vi "Write INI Cluster__ogtk.vi"(5 "float number format (optional)":string, 8 "error in (no error)":errorcluster, 10 "INI Fomatted Cluster":variant, 11 "refnum":T1) -> (0 "error out":errorcluster, 3 "dup refnum":T1)   [LabVIEW 2017]
doc: "Writes a cluster of section formatted clusters to configuration data identified by refnum. Section cluster names are used as section names and key-value pairs correspond to the named cluster elements and thier values within the section formatted clusters. Only the items within the \"INI Formatted Cluster\" input cluster are written to the configuration data.\n\nFor example an Cluster containins subClusters MyCluster1 and MyCluster2, where MyCluster1 contains two elements MyNumeric and MyBoolean, and MyCluster2 contains two elements MyEnum and MyString. This would correspond to an INI write of the following data:\n\n[MyCluster1]\nMyNumeric=1.024\nMyBoolean=TRUE\n[MyCluster2]\nMyEnum=init\nMyString=\"Hello World\"\n\nNote: Special characters in section and key names will be escape-coded. These include the following: \\00-\\1F (non-printable chars); \"[\", \"]\", and \"=\" (INI syntax elements); \\FE (\"þ\") and \\FF (\"ÿ\") (legacy bracket encoding); Additionally, the escape character, \"\\\", will be escaped as \"\\\\\".\n\nNote: This VI checks whether every element of the cluster has a name so it can be identified."
uses:
  <vilib>/Utility/config.llb/Config Data RefNum.ctl
  <vilib>/Utility/config.llb/NI_LVConfig.lvlib
panel:
  # "Write INI Cluster.vi\n\nWrites a cluster (variant) of INI section clusters to INI file.\n\nPlease visit http://www.OpenG.org to learn about the\nOpen Source LabVIEW software movement.\n\nNOTICE -- YOU MUST LEAVE THIS NOTICE IN PLACE.  PER THE TERMS OF THE LICENSE BELOW, YOU MAY SUBLICENSE THIS SOFTWARE \nIN ANY WAY THAT DOES NOT CONFLICT WITH THIS LICENSE.\n\n### BSD License (http://www.opensource.org/licenses/bsd-license.php) Begin ###\n \nCopyright (c) 2002-2006, Jim Kring <jim@jimkring.com>\n\nAll rights reserved.\n\nRedistribution and use in source and binary forms, with or without modification, are permitted provided that the following conditions are met:\n\n    * Redistributions of source code must retain the above copyright notice, this list of conditions and the following disclaimer.\n    * Redistributions in binary form must reproduce the above copyright notice, this list of conditions and the following disclaimer in the \n       documentation and/or other materials provided with the distribution.\n    * Neither the name of SciWare, James Kring, Inc., nor the names of its contributors may be used to endorse or promote products derived \n       from this software without specific prior written permission.\n\nTHIS SOFTWARE IS PROVIDED BY THE COPYRIGHT HOLDERS AND CONTRIBUTORS \"AS IS\" AND ANY EXPRESS OR IMPLIED WARRANTIES, \nINCLUDING, BUT NOT LIMITED TO, THE IMPLIED WARRANTIES OF MERCHANTABILITY AND FITNESS FOR A PARTICULAR PURPOSE ARE \nDISCLAIMED. IN NO EVENT SHALL THE COPYRIGHT OWNER OR CONTRIBUTORS BE LIABLE FOR ANY DIRECT, INDIRECT, INCIDENTAL,\n SPECIAL, EXEMPLARY, OR CONSEQUENTIAL DAMAGES (INCLUDING, BUT NOT LIMITED TO, PROCUREMENT OF SUBSTITUTE GOODS OR \nSERVICES; LOSS OF USE, DATA, OR PROFITS; OR BUSINESS INTERRUPTION) HOWEVER CAUSED AND ON ANY THEORY OF LIABILITY, \nWHETHER IN CONTRACT, STRICT LIABILITY, OR TORT (INCLUDING NEGLIGENCE OR OTHERWISE) ARISING IN ANY WAY OUT OF THE USE \nOF THIS SOFTWARE, EVEN IF ADVISED OF THE POSSIBILITY OF SUCH DAMAGE.\n\n### BSD License End ###"
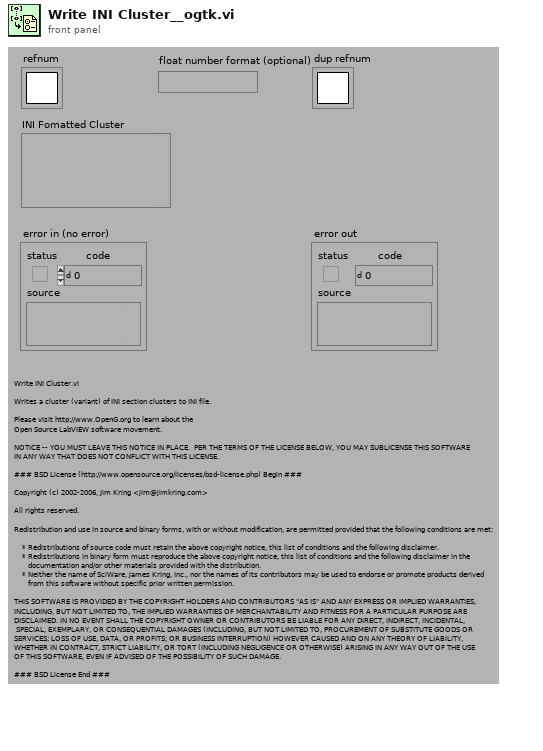
[diagram p1: front panel]
types:
  T1 = typedef "NI_LVConfig.lvlib/Config Data RefNum.ctl" = refnum<k1>
  T2 = typedef "Type Descriptor Enumeration__ogtk.ctl" = enum8{"<Null>", "I8", "I16", "I32", "I64", "U8", "U16", "U32", "U64", "SGL", "DBL", "EXT", "CSG", "CDB", "CXT", "0x0F", "0x10", "0x11", "0x12", "0x13", "0x14", "Enum U8", "Enum U16", "Enum U32", "Enum U64", "SGL PQ", "DBL PQ", "EXT PQ", "CSG PQ", "CDB PQ", "CXT PQ", "0x1F", "0x20", "Boolean", "0x22", "0x23", "0x24", "0x25", "0x26", "0x27", "0x28", "0x29", "0x2A", "0x2B", "0x2C", "0x2D", "0x2E", "0x2F", "String", "0x31", "Path", "Pict", "0x34", "0x35", "0x36", "DAQ", "0x38", "0x39", "0x3A", "0x3B", "0x3C", "0x3D", "0x3E", "0x3F", "Array", "0x41", "0x42", "0x43", "0x44", "0x45", "0x46", "0x47", "0x48", "0x49", "0x4A", "0x4B", "0x4C", "0x4D", "0x4E", "0x4F", "Cluster", "0x51", "0x52", "Variant", "Waveform", "0x55", "0x56", "0x57", "0x58", "0x59", "0x5A", "0x5B", "0x5C", "0x5D", "0x5E", "0x5F", "0x60", "0x61", "0x62", "0x63", "0x64", "0x65", "0x66", "0x67", "0x68", "0x69", "0x6A", "0x6B", "0x6C", "0x6D", "0x6E", "0x6F", "Refnum"}
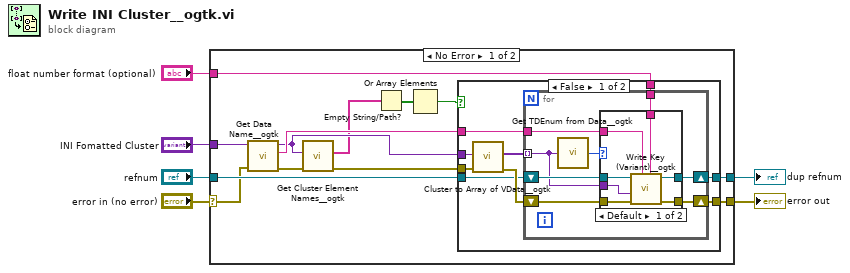
[diagram p0: block diagram]
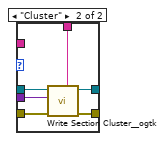
[diagram p2: hidden frame]
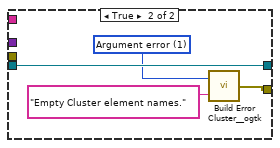
[diagram p3: hidden frame]
diagram:
  n1 = case shown="No Error" "error in (no error)" {
    selector: "error in (no error)" -> [w14 w55]
    tunnel: [w19 w55] -> w6
    tunnel: [w18 w54] -> w5
    tunnel: "refnum" -> [w17 w54]
    tunnel: "INI Fomatted Cluster" -> [w16 _]
    tunnel: "float number format (optional)" -> [w15 _]
    frame No Error {
      n2 = call <userlib>:"Get Data Name__ogtk.vi"("error in (no error)"=w14, "Data"=w16) -> ("error out"=w13:errorcluster, "Data Name"=w11:string, "Data dup"=w9:variant)  [unwired: 7 in]
      n3 = call <userlib>:"Get Cluster Element Names__ogtk.vi"("error in (no error)"=w13, "Cluster"=w9) -> ("error out"=w12:errorcluster, "Element Names"=w7:string[])  [unwired: 8 in]
      n4 = Empty String/Path?(string/path=w7) -> (empty?=w10:bool[])
      n5 = Or Array Elements(Boolean array=w10) -> (logical OR=w8:bool)
      n6 = case shown="False" w8 {
        tunnel: [w27 w52] -> w19
        tunnel: [w26 w53] -> w18
        tunnel: w17 -> [w25 w53]
        tunnel: w15 -> [w23 _]
        tunnel: w12 -> [w22 _]
        tunnel: w11 -> [w21 _]
        tunnel: w9 -> [w20 _]
        frame False {
          n7 = call <userlib>:"Cluster to Array of VData__ogtk.vi"("error in (no error)"=w22, "Cluster"=w20) -> ("error out"=w28:errorcluster, "Array of VData"=w24:variant[])  [unwired: 8 in]
          n8 = for {
            tunnel: w24 -> [w32] mode=indexing
            shift-right: [w33] -> w26
            shift-left: w25 -> [w36]
            shift-right: [w34] -> w27
            shift-left: w28 -> [w35]
            tunnel: w21 -> [w30]
            tunnel: w23 -> [w29]
            n9 = call <userlib>:"Get TDEnum from Data__ogtk.vi"("Data"=w32) -> ("Type Descriptor Enumeration"=w31:T2)  [unwired: 4 in]
            n10 = case shown="Default" w31 {
              tunnel: w36 -> [w41 w49]
              tunnel: w35 -> [w43 w48]
              tunnel: [w42 w47] -> w34
              tunnel: [w40 w46] -> w33
              tunnel: w32 -> [w38 w45]
              tunnel: w30 -> [w39 _]
              tunnel: w29 -> [w37 w44]
              frame Default {
                n11 = call <userlib>:"Write Key (Variant)__ogtk.vi"("float number format"=w37, "section"=w39, "error in (no error)"=w43, "key-value"=w38, "refnum"=w41) -> ("error out"=w42:errorcluster, "refnum out"=w40:T1)  [unwired: 5 in]
              }
              frame "Cluster" {
                n12 = call <userlib>:"Write Section Cluster__ogtk.vi"("float number format (optional)"=w44, "error in (no error)"=w48, "Section Formatted Cluster"=w45, "refnum"=w49) -> ("error out"=w47:errorcluster, "dup refnum"=w46:T1)  [unwired: 6 in]
              }
            }
          }
        }
        frame True {
          w51 = 1 items=["No error", "Argument error", "Memory is full", "Out of zone", "End of file", "File already open", "Generic file I/O error", "File not found", "File permission error", "Disk is full", "Duplicate path", "Too many files open", "System feature not enabled", "Resource file not found", "Cannot add resource", "Resource not found", "Image not found", "Image memory error", "Pen does not exist", "Config type invalid", "Config token not found", "Config parse error", "Config memory error", "Bad external code format", "Bad external code offset", "External code not present", "Null window", "Destroy window error", "Null menu", "Print aborted", "Bad print record", "Print driver error", "Windows error during printing", "Memory error during printing", "Print dialog error", "Generic print error", "Invalid device refnum", "Device not found", "Device parameter error", "Device unit error", "Cannot open device", "Device call aborted", "Generic error", "Cancelled by user", "Object ID too low", "Object ID too high", "Object not in heap", "Unknown heap", "Unknown object (invalid DefProc)", "Unknown object (DefProc not in table)", "Message out of range", "Invalid (null) method", "Unknown message", "Manager call not supported", "Bad address", "Network operation in progress", "Network operation timed out", "Connection is busy", "Network attribute not supported", "Network error", "Address in use", "System out of memory", "Connection aborted", "Connection refused", "Not connected", "Already connected", "Connection closed", "Initialization error (interapplication manager)", "Bad occurrence", "Wait on unbound occurrence handler", "Occurrence queue overflow", "Datalog type conflict", "Unused", "Unrecognized type (interapplication manager)", "Memory corrupt", "Failed to make temporary DLL", "Old CIN version", "Drag socket not found", "Failed to load drop-object", "Failed to register OLE object", "Failed to release OLE object", "Format specifier type mismatch", "Unknown format specifier", "Too few format specifiers", "Too many format specifiers", "Scan failed", "Newer CIN version", "Error converting to variant", "Runtime menu error", "Password tampered", "Variant attribute not found", "Incompatible variant data type", "Event data is not available", "Event Store is not present", "Occurrence is not found", "Event Queue is not created", "Event info is not available", "Refnum passed is NULL", "Error retrieving Class GUID", "Error retrieving CoClass GUID", "Error retrieving TypeLib GUID.", "Bad built application magic bytes.", "Specific driver is different from the specific driver associated with the Logical Name.", "There is no session opened to the class driver.", "Max Error", "MAX - Error with config objects", "MAX - Error loading configuration", "MAX - Group not supported"]
          n13 = call <userlib>:"Build Error Cluster__ogtk.vi"("String to Prepend to source (\"\")"="Empty Cluster element names." ("String to Prepend to source (\"\")"), "code"=w51) -> ("error out"=w52:errorcluster)
        }
      }
    }
    frame Error {
    }
  }
  "error out" <- w6
  "dup refnum" <- w5
